vi "ReadWriteTextFiles.vi"() -> ()   [LabVIEW 2019]
panel:
  in  "Create file here":path
  out "Read data from here":string
  in  "Provide file path here":path
  in  "Write here your own thoughts":string
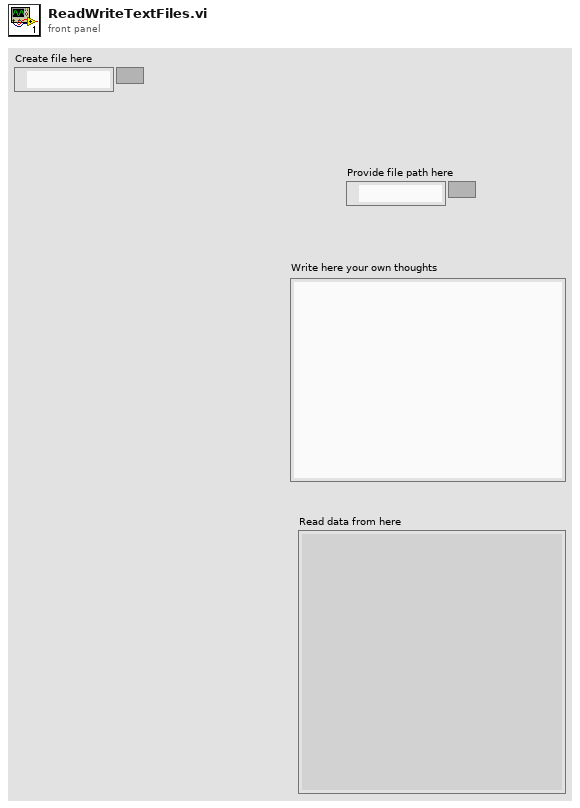
[diagram p1: front panel]
types:
  T1 = enum16{"open", "replace", "create", "open or create", "replace or create", "replace or create with confirmation"}
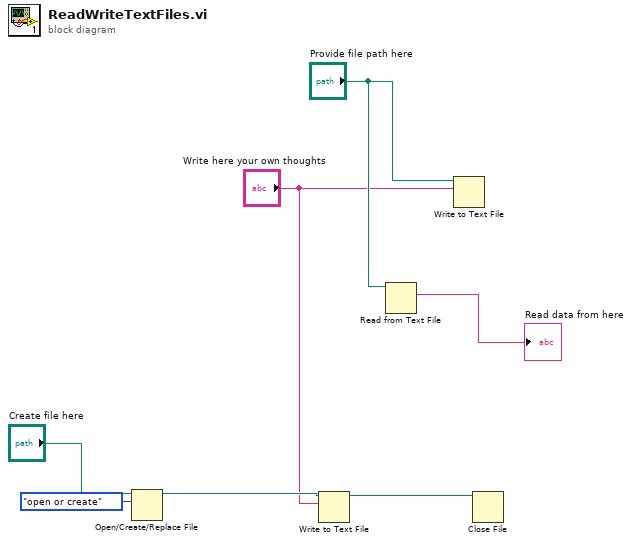
[diagram p0: block diagram]
diagram:
  n1 = Open/Create/Replace File(file path (use dialog)="Create file here", operation (0:open)=T1."open or create") -> (refnum out=w4:refnum<file>)  [unwired: 4 in, 2 out]
  n2 = Write to Text File(file (use dialog)=w4, text="Write here your own thoughts") -> (refnum out=w2:refnum<file>)  [unwired: 2 in, 2 out]
  n3 = Read from Text File(file (use dialog)="Provide file path here") -> (text=→"Read data from here":string)  [unwired: 3 in, 3 out]
  n4 = Write to Text File(file (use dialog)="Provide file path here", text="Write here your own thoughts") -> ()  [unwired: 2 in, 3 out]
  n5 = Close File(refnum=w2) -> ()  [unwired: 1 in, 2 out]
